vi "download_File.vi"(8 "error in (no error)":errorcluster, 10 "Skylink":string="TADKINn2xHrayKOwaDf5H8O8Jd8-lYiFMX4OPanGJmIh9w", 11 "Local File Path":path=path "D:/") -> (0 "error out":errorcluster)   [LabVIEW 2019, in "SiaSkynetAPI.lvlib"]
uses:
  SiaSkynetAPI.lvlib
  <vilib>/httpClient/LabVIEWHTTPClient.lvlib
panel:
  in  "portal_url":string="https://siasky.net/"
  out "headers":string="HTTP/1.1 200 OK\r\nServer: nginx/1.17.9\r\nDate: Mon, 18 May 2020 20:41:37 GMT\r\nContent-Type: application/x-msdownload\r\nContent-Length: 53157067\r\nConnection: keep-alive\r\nAccess-Control-Allow-Origin: *\r\nContent-Disposition: inline; filename=\"Sia-UI-v1.4.6.exe\"\r\nSkynet-File-Metadata: {\"filename\":\"Sia-UI-v1.4.6.exe\",\"subfiles\":{\"Sia-UI-v1.4.6.exe\":{\"filename\":\"Sia-UI-v1.4.6.exe\",\"contenttype\":\"application/x-msdownload\",\"len\":53157067}}}\r\nAccess-Control-Expose-Headers: skynet-file-metadata\r\nAccept-Ranges: bytes\r\n\r\n"
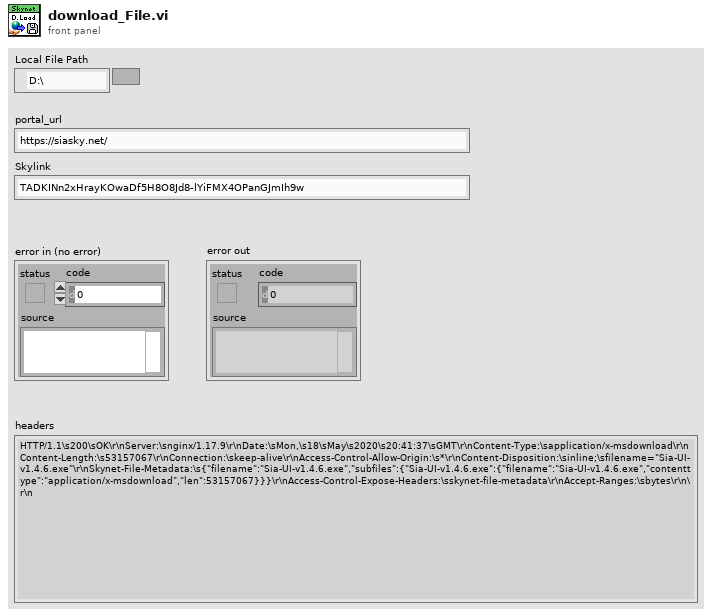
[diagram p1: front panel]
types:
  T1 = enum16{"open", "replace", "create", "open or create", "replace or create", "replace or create with confirmation"}
  T2 = typedef "LabVIEWHTTPClient.lvlib/ClientHandle.ctl" = refnum<k1>
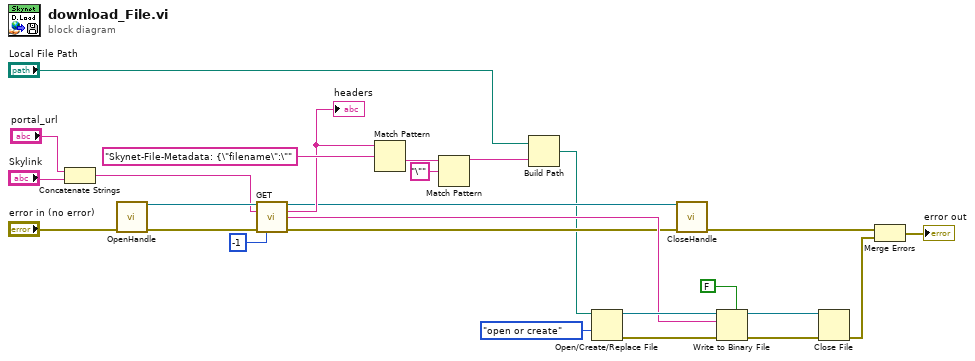
[diagram p0: block diagram]
diagram:
  n1 = Concatenate Strings("portal_url", "Skylink") -> (w2:string)
  n2 = call <vilib>:"OpenHandle.vi"("error in (no error)"="error in (no error)") -> ("client handle out"=w26:T2, "error out"=w25:errorcluster)  [unwired: 13 in]
  n3 = call <vilib>:"GET.vi"("client handle"=w26, "url"=w2, "error in (no error)"=w25, "timeout (10000)"=-1) -> ("client handle out"=w12:T2, "headers"=w16:string, "body"=w15:string, "error out"=w11:errorcluster)  [unwired: 8 in]
  "headers" <- w16
  n4 = Match Pattern(string=w16, regular expression="Skynet-File-Metadata: {\"filename\":\"" ("url")) -> (after substring=w23:string)  [unwired: 1 in, 3 out]
  n5 = Match Pattern(string=w23, regular expression="\"") -> (before substring=w21:string)  [unwired: 1 in, 3 out]
  n6 = Build Path(base path="Local File Path", name or relative path=w21) -> (appended path=w10:path)
  n7 = Open/Create/Replace File(file path (use dialog)=w10, operation (0:open)=T1."open or create") -> (refnum out=w20:refnum<file>, error out=w19:errorcluster)  [unwired: 4 in, 1 out]
  n8 = call <vilib>:"CloseHandle.vi"("client handle"=w12, "error in (no error)"=w11) -> ("error out"=w8:errorcluster)  [unwired: 13 in]
  n9 = Write to Binary File(file (use dialog)=w20, data=w15, error in=w19, 5:FALSE ("prepend array or string size? (T)")) -> (refnum out=w18:refnum<file>, error out=w17:errorcluster)  [unwired: 2 in, 1 out]
  n10 = Close File(refnum=w18, error in=w17) -> (error out=w7:errorcluster)  [unwired: 1 out]
  n11 = Merge Errors(w8, w7) -> (→"error out":errorcluster)
